vi "zadanie.vi"() -> ()   [LabVIEW 2017]
panel:
  in  "stop 2":bool
  in  "stop":bool
  out "Array 2":u32[](array[numeric])
  out "Array":u32[](array[numeric])
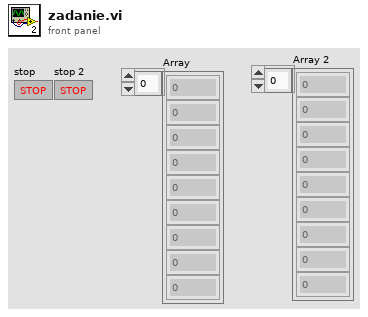
[diagram p1: front panel]
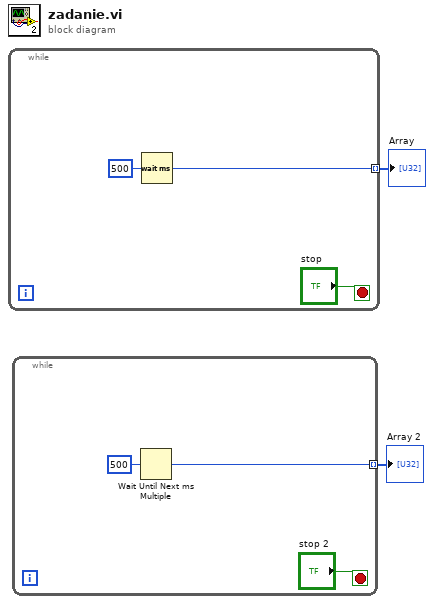
[diagram p0: block diagram]
diagram:
  n1 = while {
    tunnel: [w4] -> w2 mode=indexing
    stop <- "stop" stop-if-true
    n2 = Wait (ms)(milliseconds to wait=u32 500) -> (millisecond timer value=w4:u32)
  }
  "Array" <- w2
  n3 = while {
    tunnel: [w7] -> w1 mode=indexing
    stop <- "stop 2" stop-if-true
    n4 = Wait Until Next ms Multiple(millisecond multiple=u32 500) -> (millisecond timer value=w7:u32)
  }
  "Array 2" <- w1
